vi "PlotIntensityGraph.vi"(0 "IntensityGraph in":refnum<vi>, 1 "System no.":i32, 2 "Mesh":dbl, 3 "Lower thr":dbl, 4 "X Scan Range":dbl, 5 "error in (no error)":errorcluster, 6 "Map centers":dbl[](array[numeric]), 7 "Y Scan Range":dbl, 9 "Upper thr":dbl) -> (10 "Xoffset":dbl, 12 "Yoffset":dbl, 13 "Plot Images:Front":picture, 14 "Array":dbl[][](array[numeric]), 15 "cent":i32[][](array[numeric]), 16 "Numeric":i32, 17 "Intensity Graph":dbl[][](array[numeric]), 18 "Nemitters":i32, 19 "error out":errorcluster)   [LabVIEW 2023]
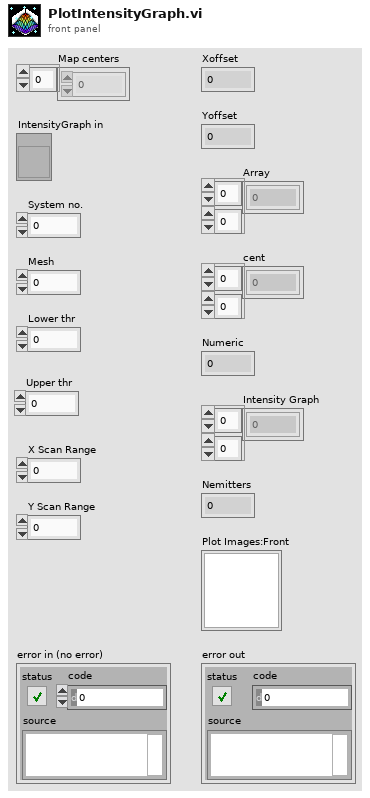
[diagram p1: front panel]
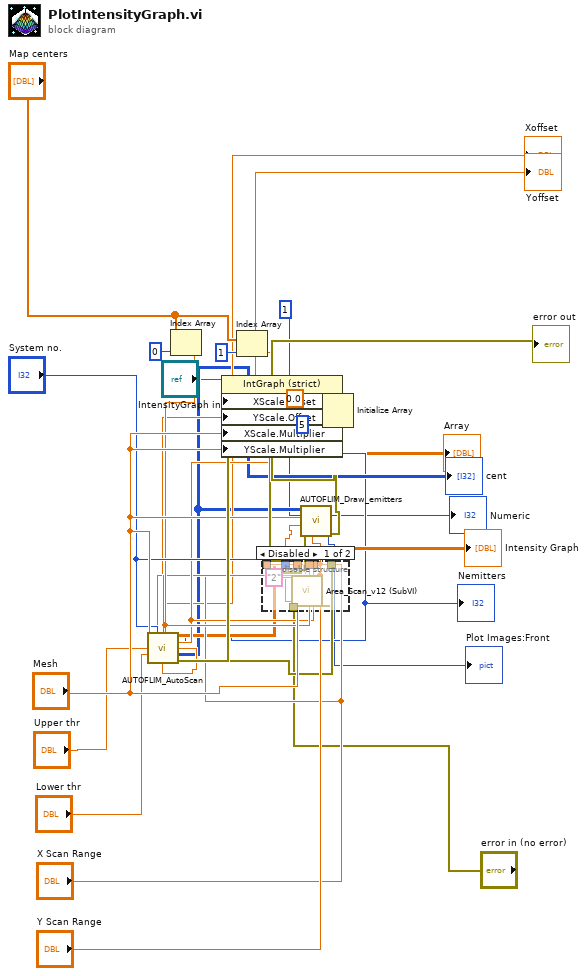
[diagram p0: block diagram]
diagram:
  n1 = Index Array(array="Map centers", index=0) -> (element=w22:dbl)
  n2 = Index Array(array="Map centers", index=1) -> (element=w21:dbl)
  n3 = disable-structure shown="Disabled" {
    disable-tunnel: "error in (no error)" -> [w36 _]
    disable-tunnel: [w35 _] -> w18
    disable-tunnel: "X Scan Range" -> [w34 _]
    disable-tunnel: "Y Scan Range" -> [w33 _]
    disable-tunnel: w21 -> [w32 _]
    disable-tunnel: w22 -> [w31 _]
    disable-tunnel: "System no." -> [w29 _]
    disable-tunnel: "Mesh" -> [w28 _]
    frame Disabled {
      n4 = call "Area_Scan_v12 (SubVI).vi"("Step Axis"="2", "System no."=w29, "error in (no error)"=w36, "Mesh in"=w28, "X Scan Range"=w34, "Y Scan Range"=w33, "X Scan Center"=w31, "Y Scan Center"=w32) -> ("error out"=w35:errorcluster)  [unwired: 15 in, 4 out]
    }
    frame Enabled {
    }
  }
  n5 = call "AUTOFLIM_AutoScan.vi"("X Scan Center"=w22, "System#"="System no.", "Mesh"="Mesh", "Y Scan Center"=w21, "Upper thr"="Upper thr", "Lower Thr"="Lower thr", "error in (no error)"=w18, "X Scan Range"="X Scan Range", "Y Scan Range"="Y Scan Range") -> ("Xoffset"=w12:dbl, "Intensity Graph"=→"Intensity Graph":dbl[][], "Nemitters"=w9:i32, "Yoffset"=w13:dbl, "cent"=w10:i32[][], "error out"=w25:errorcluster)  [unwired: 1 in]
  "Yoffset" <- w13
  "Xoffset" <- w12
  "cent" <- w10
  "Nemitters" <- w9
  n6 = property on="Property Node" class="IntGraph (strict)"(reference="IntensityGraph in", error in=w25, "XScale.Offset"=w12, "YScale.Offset"=w13, "XScale.Multiplier"="Mesh", "YScale.Multiplier"="Mesh") -> (error out=w26:errorcluster)  [unwired: 1 out]
  n7 = call "AUTOFLIM_Draw_emitters.vi"("Y Scan Range"="Y Scan Range", "error in (no error)"=w26, "X Scan Range"="X Scan Range", "Mesh"="Mesh", "cent"=w10) -> ("error out"=→"error out":errorcluster, "Plot Images:Front"=→"Plot Images:Front":picture)  [unwired: 5 in]
  n8 = Initialize Array(0.0 ("element"), w9, 5 ("dimension size")) -> (→"Array":dbl[][])
  "Numeric" <- 1
